vi "PrepareFirmware.vi"(1 "Firmware file":path) -> (0 "Firmware data":string[](array[string]))   [LabVIEW 2010]
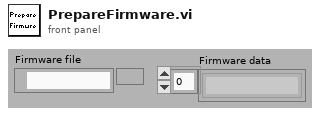
[diagram p1: front panel]
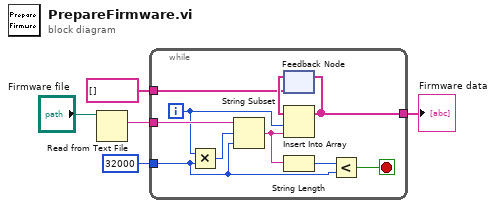
[diagram p0: block diagram]
diagram:
  n1 = Read from Text File(file (use dialog)="Firmware file") -> (text=w5:string)  [unwired: 3 in, 3 out]
  n2 = while {
    tunnel: w5 -> [w15]
    tunnel: 32000 -> [w12]
    tunnel: string[] [] -> [w7]
    tunnel: [w6] -> w1
    i -> [w10]
    stop <- w11 stop-if-true
    n3 = Multiply(x=w10, y=w12) -> (x*y=w14:i32)
    n4 = String Subset(string=w15, offset (0)=w14, length (rest)=w12) -> (substring=w9:string)
    n5 = feedback #1(w7) -> (w8:string[])
    n6 = Insert Into Array(array=w8, index=w10, new element=w9) -> (w6:string[])
    n7 = feedback-in #1(w6) -> ()
    n8 = String Length(string=w9) -> (length=w13:i32)
    n9 = Less?(x=w13, y=w12) -> (x < y?=w11:bool)
  }
  "Firmware data" <- w1
